vi "clean_delay_channels.vi"(11 "Ramp Delay Settings":T1={"Insert Delays"=FALSE, "Number of loops"=0, "Insert after instruction"=0, "Random"=FALSE, "Initial Delay Time (s)"=0.0, "Final Delay Time (s)"=5e-08, "Delay Step (s)"=5e-08, "Delay Column"=0.0, "Loop Hold Column"=0.0, "Field Ramp Column"=0.0, "Excitation Column"=0.0, "Hold + Delay + Excitation Time"=0.0, "Ascending/Descending"=FALSE, "Subroutine A"=[{"Instruct Data"=0, "Op Code"=0, "Flags"=[FALSE, TRUE, TRUE, TRUE, FALSE, TRUE, TRUE, TRUE, FALSE, FALSE, FALSE, TRUE, TRUE, FALSE, FALSE, FALSE, TRUE, FALSE, FALSE, FALSE, FALSE, FALSE, TRUE, FALSE], "Comments"="Loop hold", "Time (s)"=1e-05, "Column Number"="", "Array"=[]}, {"Instruct Data"=0, "Op Code"=0, "Flags"=[FALSE, FALSE, TRUE, FALSE, FALSE, TRUE, TRUE, TRUE, FALSE, FALSE, FALSE, TRUE, TRUE, FALSE, FALSE, FALSE, TRUE, FALSE, FALSE, FALSE, FALSE, FALSE, TRUE, FALSE], "Comments"="Expose UV", "Time (s)"=0.081, "Column Number"="", "Array"=[]}, {"Instruct Data"=0, "Op Code"=0, "Flags"=[FALSE, TRUE, TRUE, TRUE, FALSE, TRUE, TRUE, TRUE, FALSE, FALSE, FALSE, TRUE, TRUE, FALSE, FALSE, FALSE, TRUE, FALSE, FALSE, FALSE, FALSE, FALSE, TRUE, FALSE], "Comments"="Hold Rydbies", "Time (s)"=1e-05, "Column Number"="", "Array"=[]}, {"Instruct Data"=0, "Op Code"=6, "Flags"=[FALSE, FALSE, FALSE, FALSE, FALSE, TRUE, TRUE, TRUE, FALSE, FALSE, FALSE, FALSE, TRUE, FALSE, FALSE, FALSE, TRUE, FALSE, FALSE, FALSE, FALSE, FALSE, TRUE, FALSE], "Comments"="Count", "Time (s)"=0.5, "Column Number"="", "Array"=[]}]} {"Subroutine A"."Time (s)" min=5e-08 format="%.2p"; "Subroutine A"."Op Code" items=["Continue", "Stop", "Loop", "End Loop", "JSR", "RTS", "Go To", "Long Delay", "Wait"]; "Subroutine A"."Instruct Data" format="%#.2p"; "Delay Column" min=5e-08 format="%#_6p"; "Delay Step (s)" min=5e-08 format="%#_6p"; "Final Delay Time (s)" min=5e-08 format="%#_6p"; "Initial Delay Time (s)" min=5e-08 format="%#_6p"}) -> (3 "Ramp Delay Settings Out":T1={"Insert Delays"=FALSE, "Number of loops"=0, "Insert after instruction"=0, "Random"=FALSE, "Initial Delay Time (s)"=0.0, "Final Delay Time (s)"=5e-08, "Delay Step (s)"=5e-08, "Delay Column"=0.0, "Loop Hold Column"=0.0, "Field Ramp Column"=0.0, "Excitation Column"=0.0, "Hold + Delay + Excitation Time"=0.0, "Ascending/Descending"=FALSE, "Subroutine A"=[{"Instruct Data"=0, "Op Code"=0, "Flags"=[FALSE, TRUE, TRUE, TRUE, FALSE, TRUE, TRUE, TRUE, FALSE, FALSE, FALSE, TRUE, TRUE, FALSE, FALSE, FALSE, TRUE, FALSE, FALSE, FALSE, FALSE, FALSE, TRUE, FALSE], "Comments"="Loop hold", "Time (s)"=1e-05, "Column Number"="", "Array"=[]}, {"Instruct Data"=0, "Op Code"=0, "Flags"=[FALSE, FALSE, TRUE, FALSE, FALSE, TRUE, TRUE, TRUE, FALSE, FALSE, FALSE, TRUE, TRUE, FALSE, FALSE, FALSE, TRUE, FALSE, FALSE, FALSE, FALSE, FALSE, TRUE, FALSE], "Comments"="Expose UV", "Time (s)"=0.081, "Column Number"="", "Array"=[]}, {"Instruct Data"=0, "Op Code"=0, "Flags"=[FALSE, TRUE, TRUE, TRUE, FALSE, TRUE, TRUE, TRUE, FALSE, FALSE, FALSE, TRUE, TRUE, FALSE, FALSE, FALSE, TRUE, FALSE, FALSE, FALSE, FALSE, FALSE, TRUE, FALSE], "Comments"="Hold Rydbies", "Time (s)"=1e-05, "Column Number"="", "Array"=[]}, {"Instruct Data"=0, "Op Code"=6, "Flags"=[FALSE, FALSE, FALSE, FALSE, FALSE, TRUE, TRUE, TRUE, FALSE, FALSE, FALSE, FALSE, TRUE, FALSE, FALSE, FALSE, TRUE, FALSE, FALSE, FALSE, FALSE, FALSE, TRUE, FALSE], "Comments"="Count", "Time (s)"=0.5, "Column Number"="", "Array"=[]}]} {"Subroutine A"."Time (s)" min=5e-08 format="%.2p"; "Subroutine A"."Op Code" items=["Continue", "Stop", "Loop", "End Loop", "JSR", "RTS", "Go To", "Long Delay", "Wait"]; "Subroutine A"."Instruct Data" format="%#.2p"; "Delay Column" min=5e-08 format="%#_6p"; "Delay Step (s)" min=5e-08 format="%#_6p"; "Final Delay Time (s)" min=5e-08 format="%#_6p"; "Initial Delay Time (s)" min=5e-08 format="%#_6p"})   [LabVIEW 2016]
uses:
  Controls/PulseBlaster/delay_control_3..ctl
  Controls/PulseBlaster/Instructions_Cluster.ctl
  Controls/PulseBlaster/24ch_single_timing_column.ctl
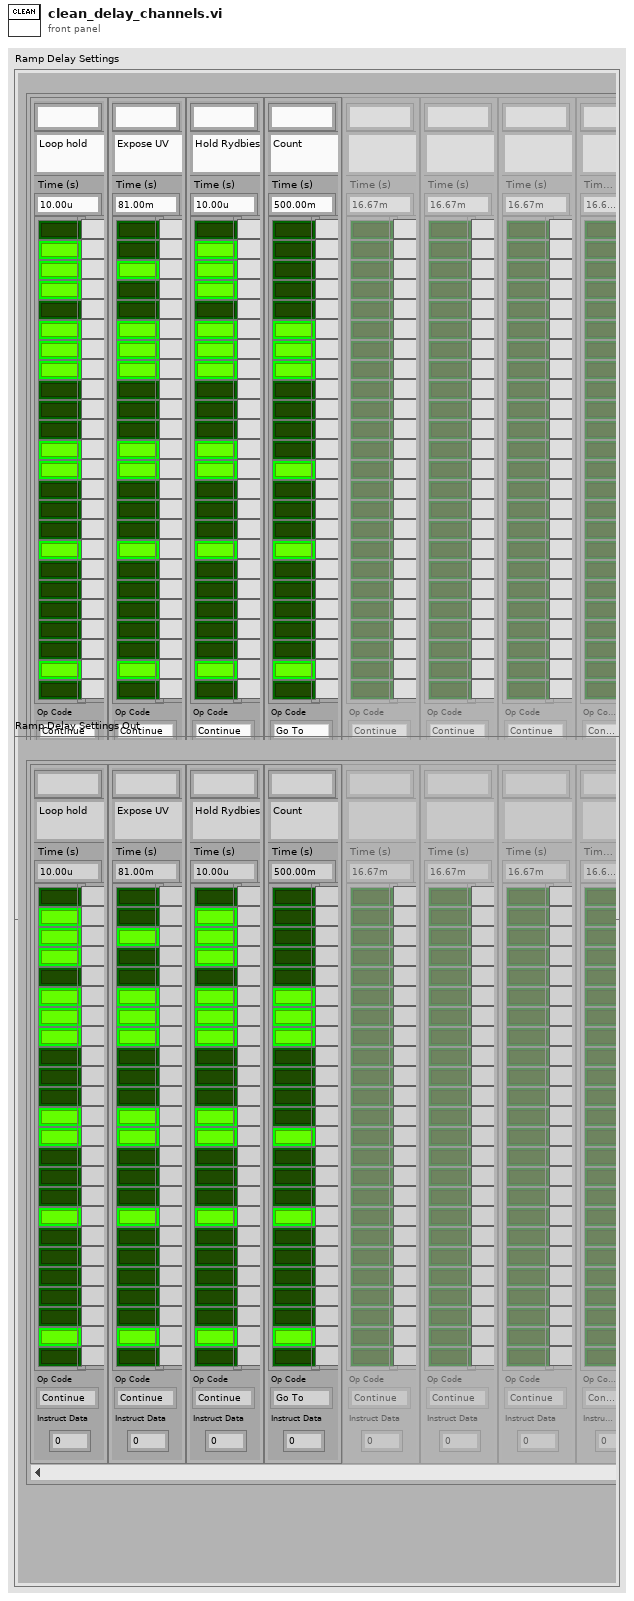
[diagram p1: front panel]
types:
  T1 = typedef "delay_control_3..ctl" = cluster{"Insert Delays":bool, "Number of loops":i32, "Insert after instruction":i32, "Random":bool, "Initial Delay Time (s)":dbl, "Final Delay Time (s)":dbl, "Delay Step (s)":dbl, "Delay Column":dbl, "Loop Hold Column":dbl, "Field Ramp Column":dbl, "Excitation Column":dbl, "Hold + Delay + Excitation Time":dbl, "Ascending/Descending":bool, "Subroutine A":T2}
  T2 = typedef "Instructions_Cluster.ctl" = T3[]
  T3 = typedef "24ch_single_timing_column.ctl" = cluster{"Instruct Data":i32, "Op Code":i32, "Flags":bool[], "Comments":string, "Time (s)":dbl, "Column Number":string, "Array":string[]}
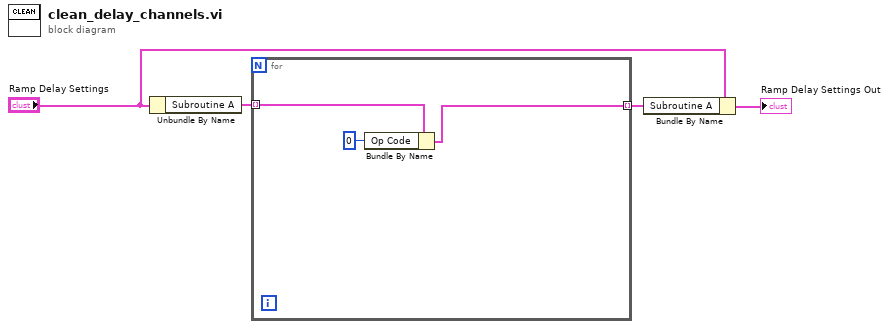
[diagram p0: block diagram]
diagram:
  n1 = Unbundle By Name("Ramp Delay Settings") -> ("Subroutine A"=w4:T2)
  n2 = for {
    tunnel: w4 -> [w7] mode=indexing
    tunnel: [w5] -> w3 mode=indexing
    n3 = Bundle By Name(cluster=w7, "Op Code"=0) -> (w5:T3)
  }
  n4 = Bundle By Name(cluster="Ramp Delay Settings", "Subroutine A"=w3) -> (→"Ramp Delay Settings Out":T1)
